vi "Find FPGA Addon Custom Devices.vi"(8 "error in (no error)":errorcluster, 11 "target in":refnum<k24>) -> (0 "error out":errorcluster, 1 "found ?":bool, 2 "FPGA Addon refnums out":T1[](array[typedef]) format="%.0x", 3 "target out":refnum<k24>)   [LabVIEW 2018, in "Scripting API.lvlib"]
uses:
  Scripting API.lvlib
  NationalInstruments.VeriStand.SystemDefinitionAPI
  <vilib>/NI Veristand/Custom Device API/Custom Device Item Ref.ctl
  Addon/Addon Shared/SubVIs/Constants.vi
  <vilib>/NI Veristand/Custom Device API/Custom Device API.lvlib
  Addon/Addon Shared/FPGA Addon Shared.lvlib
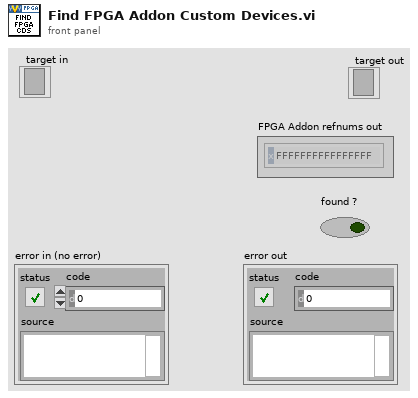
[diagram p1: front panel]
types:
  T1 = typedef "Custom Device API.lvlib/Custom Device Item Ref.ctl" = u64
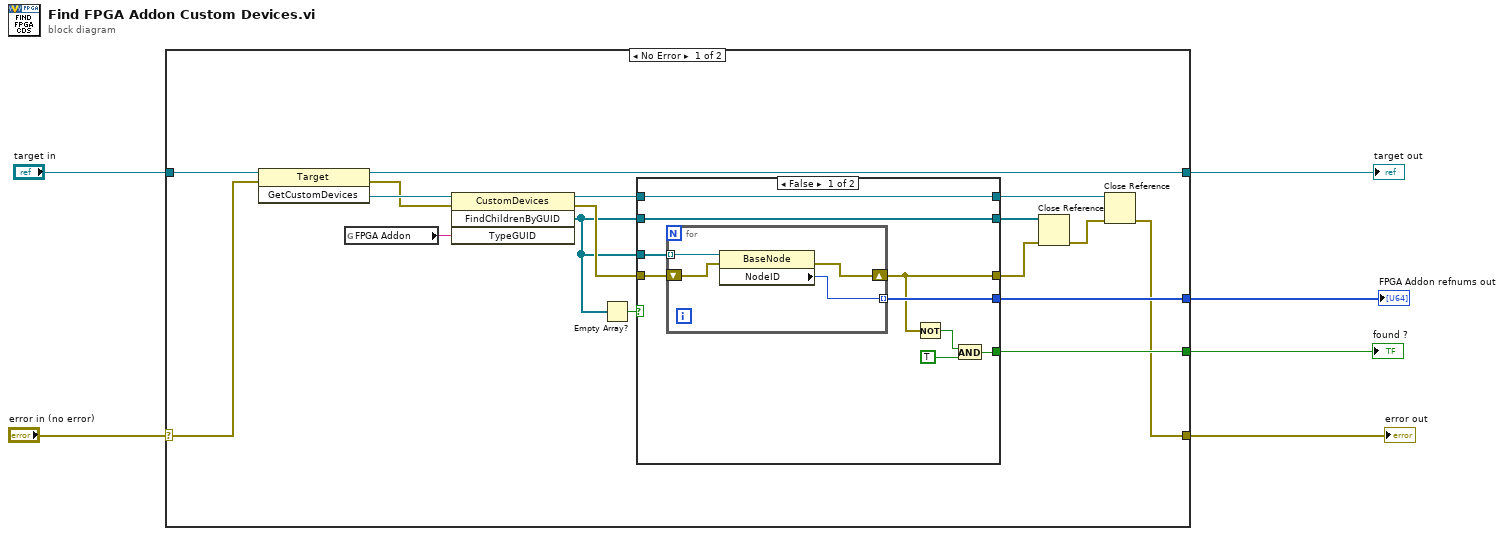
[diagram p0: block diagram]
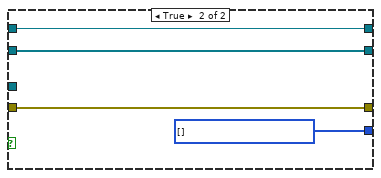
[diagram p2: hidden frame]
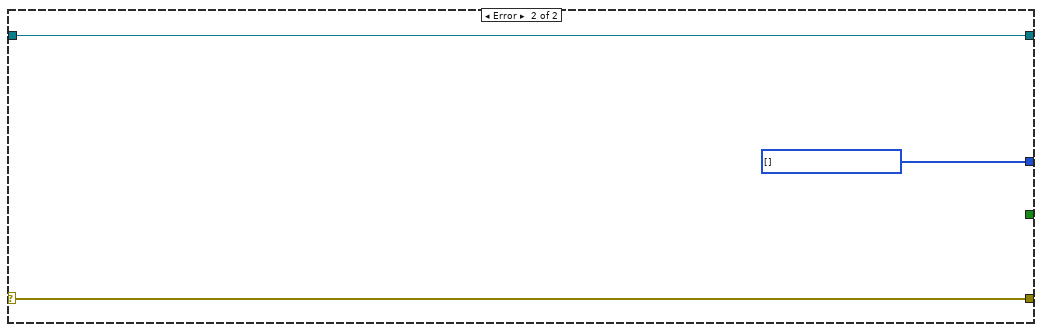
[diagram p3: hidden frame]
diagram:
  n1 = case shown="No Error" "error in (no error)" {
    selector: "error in (no error)" -> [w21 w43]
    tunnel: [w23 w41] -> w5
    tunnel: [w7 w43] -> w1
    tunnel: [w18 _] -> w4
    tunnel: [w14 T1[] []] -> w6
    tunnel: "target in" -> [w13 w41]
    frame No Error {
      n2 = invoke class="Target" method="GetCustomDevices"(reference=w13, error in=w21) -> (reference out=w23:refnum<k24>, error out=w20:errorcluster, "GetCustomDevices"=w22:refnum<k24>)  [unwired: 1 in]
      n3 = global read "Constants.vi" "FPGA Addon"() -> (w16:string)
      n4 = invoke class="CustomDevices" method="FindChildrenByGUID"(reference=w22, error in=w20, "TypeGUID"=w16) -> (reference out=w17:refnum<k24>, error out=w19:errorcluster, "FindChildrenByGUID"=w12:refnum<k24>[])  [unwired: 1 in, 1 out]
      n5 = Empty Array?(array=w12) -> (empty?=w15:bool)
      n6 = case shown="False" w15 {
        tunnel: w19 -> [w32 w40]
        tunnel: [w25 w40] -> w11
        tunnel: [w24 _] -> w18
        tunnel: w17 -> [w28 w39]
        tunnel: w12 -> [w31 _]
        tunnel: [w30 T1[] []] -> w14
        tunnel: w12 -> [w29 w38]
        tunnel: [w29 w38] -> w10
        tunnel: [w28 w39] -> w9
        frame False {
          n7 = for {
            shift-right: [w35] -> w25
            shift-left: w32 -> [w36]
            tunnel: w31 -> [w34] mode=indexing
            tunnel: [w33] -> w30 mode=indexing
            n8 = property class="BaseNode"(reference=w34, error in=w36) -> (error out=w35:errorcluster, "NodeID"=w33:u64)  [unwired: 1 out]
          }
          n9 = Not(x=w25) -> (.not. x?=w26:bool)
          n10 = And(x=w26, y=TRUE) -> (x .and. y?=w24:bool)
        }
        frame True {
        }
      }
      n11 = Close Reference(reference=w10, error in (no error)=w11) -> (error out=w8:errorcluster)
      n12 = Close Reference(reference=w9, error in (no error)=w8) -> (error out=w7:errorcluster)
    }
    frame Error {
    }
  }
  "target out" <- w5
  "error out" <- w1
  "found ?" <- w4
  "FPGA Addon refnums out" <- w6
